vi "_CSM Scripts Colors.vi"(8 "Error In":errorcluster caption="error in (no error)", 11 "Value":string) -> (0 "error out":errorcluster, 3 "Array":T1(array[cluster]))   [LabVIEW 2017]
uses:
  _Shared/CSM Shared.lvlib
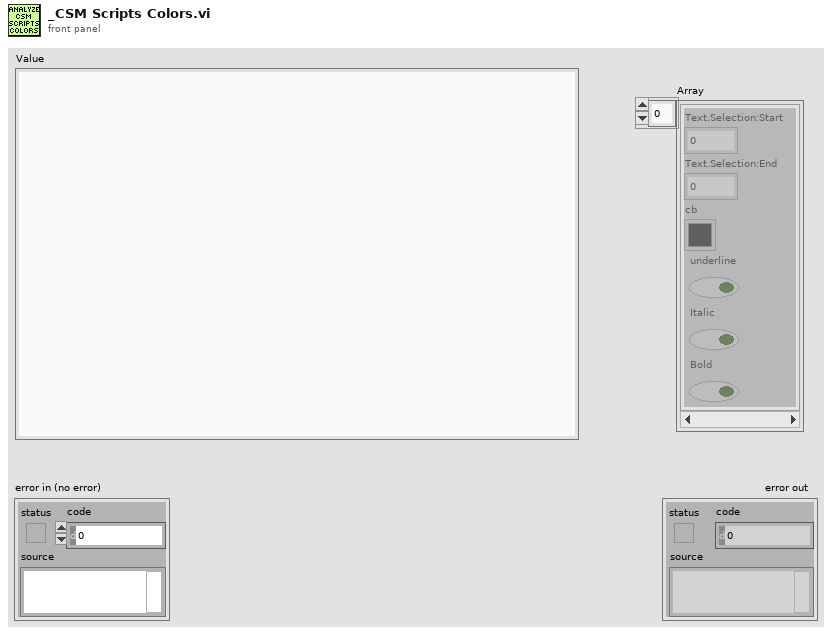
[diagram p1: front panel]
types:
  T1 = cluster{"Text.Selection:Start":u32, "Text.Selection:End":u32, "cb":u32, "underline":bool, "Italic":bool, "Bold":bool}[]
  T2 = cluster{"Text.Selection:Start":u32, u32, u32, bool, bool, bool}
  T3 = cluster{"Text.Selection:Start":u32, u32, u32, bool, bool, bool}[]
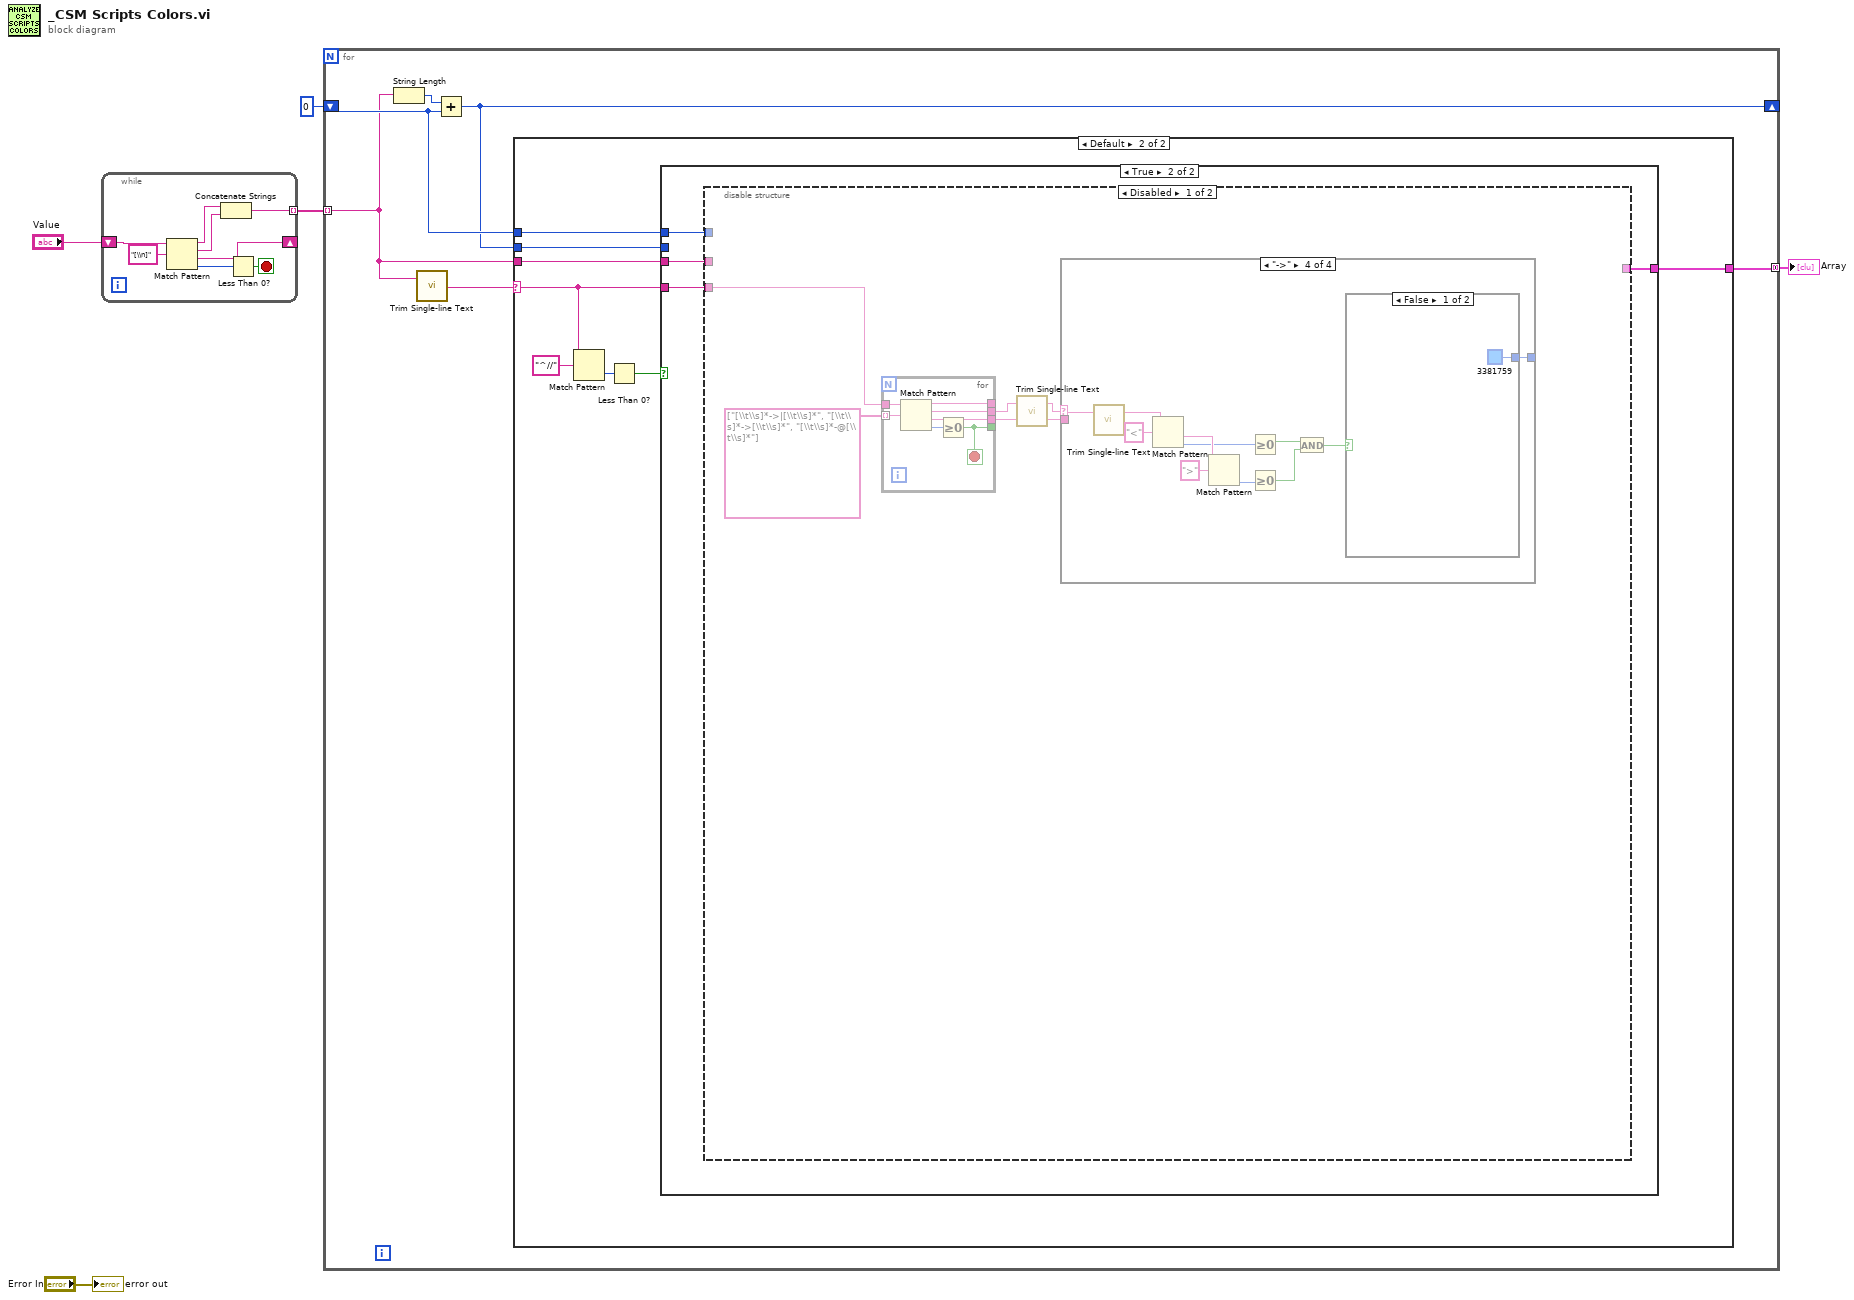
[diagram p0: block diagram]
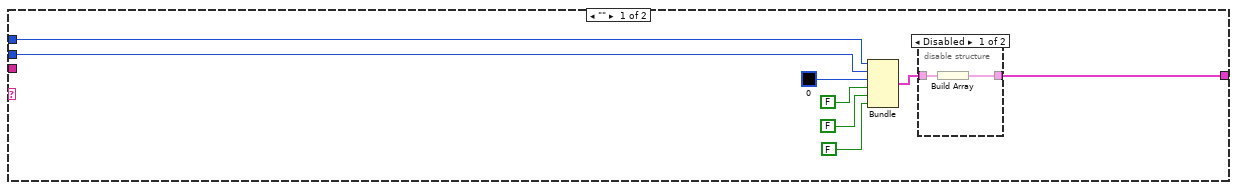
[diagram p2: hidden frame]
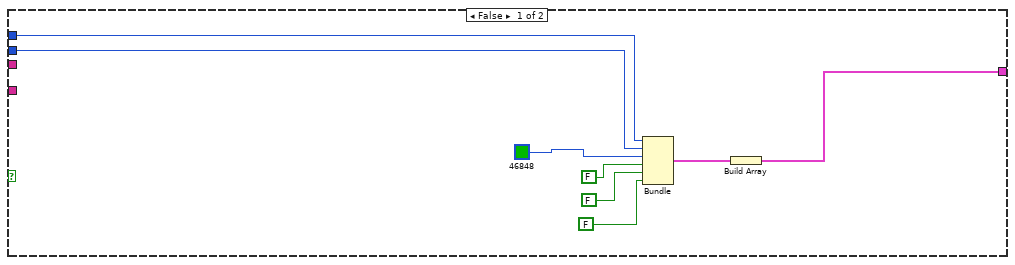
[diagram p4: hidden frame]
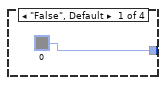
[diagram p5: hidden frame]
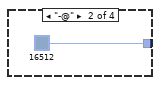
[diagram p6: hidden frame]
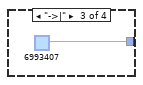
[diagram p7: hidden frame]
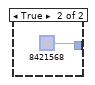
[diagram p8: hidden frame]
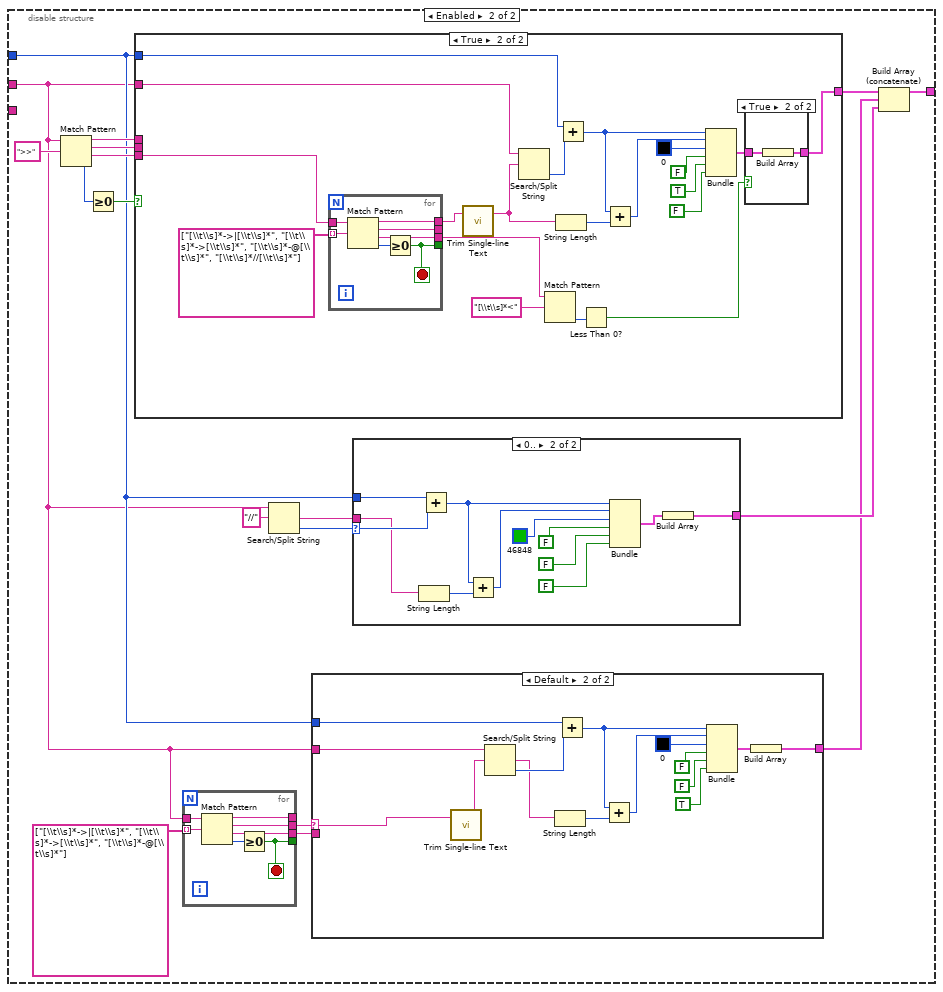
[diagram p9: hidden frame]
diagram:
  n1 = while {
    shift-right: [w12] -> _
    shift-left: "Value" -> [w13]
    tunnel: [w8] -> w5 mode=indexing
    stop <- w6 stop-if-true
    n2 = Match Pattern(string=w13, regular expression="[\\n]") -> (before substring=w10:string, match substring=w9:string, after substring=w12:string, offset past match=w7:i32)  [unwired: 1 in]
    n3 = Concatenate Strings(w10, w9) -> (w8:string)
    n4 = Less Than 0?(x=w7) -> (x < 0?=w6:bool)
  }
  n5 = for {
    tunnel: w5 -> [w14] mode=indexing
    shift-right: [w16] -> _
    shift-left: u32 0 ("Text.Selection:Start") -> [w17]
    tunnel: [w15] -> w2 mode=concatenating
    n6 = String Length(string=w14) -> (length=w18:i32)
    n7 = call "Trim Single-line Text.vi"("single-line text"=w14) -> ("trimed text"=w19:string)  [unwired: 2 in]
    n8 = Add(x=w18, y=w17) -> (x+y=w16:u32)
    n9 = case shown="Default" w19 {
      selector: w19 -> [_ w35]
      tunnel: w17 -> [w27 w32]
      tunnel: w16 -> [w26 w31]
      tunnel: [w23 w30] -> w15
      tunnel: w14 -> [_ w33]
      frame "" {
        n10 = Bundle("Text.Selection:Start"=w27, w26, u32 0, FALSE, FALSE, FALSE) -> (w24:T2)  [unwired: 1 in]
        n11 = disable-structure shown="Disabled" {
          disable-tunnel: w24 -> [w29 _]
          disable-tunnel: [w28 _] -> w23
          frame Disabled {
            n12 = Build Array(w29) -> (w28:T3)
          }
          frame Enabled {
          }
        }
      }
      frame Default {
        n13 = Match Pattern(string=w35, regular expression="^//") -> (offset past match=w37:i32)  [unwired: 1 in, 3 out]
        n14 = Less Than 0?(x=w37) -> (x < 0?=w34:bool)
        n15 = case shown="True" w34 {
          tunnel: w35 -> [_ w49]
          tunnel: w33 -> [_ w48]
          tunnel: w32 -> [w44 w47]
          tunnel: w31 -> [w43 _]
          tunnel: [w41 w46] -> w30
          frame False {
            n16 = Bundle("Text.Selection:Start"=w44, w43, u32 46848, FALSE, FALSE, FALSE) -> (w42:T2)  [unwired: 1 in]
            n17 = Build Array(w42) -> (w41:T3)
          }
          frame True {
            n18 = disable-structure shown="Disabled" {
              disable-tunnel: w49 -> [w52 _]
              disable-tunnel: w48 -> [_ w78]
              disable-tunnel: w47 -> [_ w81]
              disable-tunnel: [_ w85] -> w46
              frame Disabled {
                n19 = for {
                  tunnel: w52 -> [w77]
                  tunnel: string[] ["[\\t\\s]*->|[\\t\\s]*", "[\\t\\s]*->[\\t\\s]*", "[\\t\\s]*-@[\\t\\s]*"] -> [w76] mode=indexing
                  tunnel: [w74] -> _
                  tunnel: [w73] -> _
                  tunnel: [w72] -> w53
                  tunnel: [w71] -> w50
                  stop <- w74 stop-if-true
                  n20 = Match Pattern(string=w77, regular expression=w76) -> (before substring=w73:string, match substring=w72:string, after substring=w71:string, offset past match=w75:i32)  [unwired: 1 in]
                  n21 = Greater Or Equal To 0?(x=w75) -> (x >= 0?=w74:bool)
                }
                n22 = call "Trim Single-line Text.vi"("single-line text"=w53) -> ("trimed text"=w51:string)  [unwired: 2 in]
                n23 = case shown="\"->\"" w51 {
                  tunnel: [u32 0 u32 16512 u32 6993407 w68] -> _
                  tunnel: w50 -> [_ _ _ w67]
                  frame "False", Default {
                  }
                  frame "-@" {
                  }
                  frame "->|" {
                  }
                  frame "->" {
                    n24 = call "Trim Single-line Text.vi"("single-line text"=w67) -> ("trimed text"=w66:string)  [unwired: 2 in]
                    n25 = Match Pattern(string=w66, regular expression="<") -> (after substring=w63:string, offset past match=w61:i32)  [unwired: 1 in, 2 out]
                    n26 = Match Pattern(string=w63, regular expression=">") -> (offset past match=w62:i32)  [unwired: 1 in, 3 out]
                    n27 = Greater Or Equal To 0?(x=w61) -> (x >= 0?=w60:bool)
                    n28 = Greater Or Equal To 0?(x=w62) -> (x >= 0?=w59:bool)
                    n29 = And(x=w60, y=w59) -> (x .and. y?=w58:bool)
                    n30 = case shown="False" w58 {
                      tunnel: [u32 3381759 u32 8421568] -> w68
                      frame False {
                      }
                      frame True {
                      }
                    }
                  }
                }
              }
              frame Enabled {
                n31 = Match Pattern(string=w78, regular expression=">>") -> (before substring=w94:string, match substring=w95:string, after substring=w91:string, offset past match=w92:i32)  [unwired: 1 in]
                n32 = Greater Or Equal To 0?(x=w92) -> (x >= 0?=w93:bool)
                n33 = case shown="True" w93 {
                  tunnel: w91 -> [_ w149]
                  tunnel: w94 -> [_ _]
                  tunnel: w95 -> [_ _]
                  tunnel: w78 -> [_ w147]
                  tunnel: w81 -> [_ w145]
                  tunnel: [_ w137] -> w89
                  frame False {
                  }
                  frame True {
                    n34 = for {
                      tunnel: w149 -> [w158]
                      tunnel: string[] ["[\\t\\s]*->|[\\t\\s]*", "[\\t\\s]*->[\\t\\s]*", "[\\t\\s]*-@[\\t\\s]*", "[\\t\\s]*//[\\t\\s]*"] -> [w157] mode=indexing
                      tunnel: [w155] -> _
                      tunnel: [w154] -> w142
                      tunnel: [w153] -> _
                      tunnel: [w152] -> w134
                      stop <- w155 stop-if-true
                      n35 = Match Pattern(string=w158, regular expression=w157) -> (before substring=w154:string, match substring=w153:string, after substring=w152:string, offset past match=w156:i32)  [unwired: 1 in]
                      n36 = Greater Or Equal To 0?(x=w156) -> (x >= 0?=w155:bool)
                    }
                    n37 = call "Trim Single-line Text.vi"("single-line text"=w142) -> ("trimed text"=w130:string)  [unwired: 2 in]
                    n38 = Search/Split String(string=w147, search string/char (-)=w130) -> (offset of match=w146:i32)  [unwired: 1 in, 2 out]
                    n39 = Match Pattern(string=w134, regular expression="[\\t\\s]*<") -> (offset past match=w132:i32)  [unwired: 1 in, 3 out]
                    n40 = String Length(string=w130) -> (length=w141:i32)
                    n41 = Add(x=w145, y=w146) -> (x+y=w140:u32)
                    n42 = Less Than 0?(x=w132) -> (x < 0?=w131:bool)
                    n43 = Add(x=w140, y=w141) -> (x+y=w139:u32)
                    n44 = Bundle(w140, w139, u32 0, FALSE, TRUE, FALSE) -> (w138:cluster{u32, u32, u32, bool, bool, bool})  [unwired: 1 in]
                    n45 = case shown="True" w131 {
                      tunnel: w138 -> [_ w151]
                      tunnel: [_ w150] -> w137
                      frame False {
                      }
                      frame True {
                        n46 = Build Array(w151) -> (w150:cluster{u32, u32, u32, bool, bool, bool}[])
                      }
                    }
                  }
                }
                n47 = for {
                  tunnel: w78 -> [w117]
                  tunnel: string[] ["[\\t\\s]*->|[\\t\\s]*", "[\\t\\s]*->[\\t\\s]*", "[\\t\\s]*-@[\\t\\s]*"] -> [w116] mode=indexing
                  tunnel: [w114] -> _
                  tunnel: [w113] -> _
                  tunnel: [w112] -> w82
                  tunnel: [w111] -> w79
                  stop <- w114 stop-if-true
                  n48 = Match Pattern(string=w117, regular expression=w116) -> (before substring=w113:string, match substring=w112:string, after substring=w111:string, offset past match=w115:i32)  [unwired: 1 in]
                  n49 = Greater Or Equal To 0?(x=w115) -> (x >= 0?=w114:bool)
                }
                n50 = Search/Split String(string=w78, search string/char (-)="//" ("regular expression")) -> (match + rest of string=w86:string, offset of match=w87:i32)  [unwired: 1 in, 1 out]
                n51 = case shown="Default" w82 {
                  selector: w82 -> [_ w100]
                  tunnel: w78 -> [_ w101]
                  tunnel: w81 -> [_ w97]
                  tunnel: [_ w96] -> w80
                  tunnel: w79 -> [_ _]
                  frame "" {
                  }
                  frame Default {
                    n52 = call "Trim Single-line Text.vi"("single-line text"=w100) -> ("trimed text"=w99:string)  [unwired: 2 in]
                    n53 = Search/Split String(string=w101, search string/char (-)=w99) -> (match + rest of string=w98:string, offset of match=w110:i32)  [unwired: 1 in, 1 out]
                    n54 = String Length(string=w98) -> (length=w107:i32)
                    n55 = Add(x=w97, y=w110) -> (x+y=w106:u32)
                    n56 = Add(x=w106, y=w107) -> (x+y=w105:u32)
                    n57 = Bundle(w106, w105, u32 0, FALSE, FALSE, TRUE) -> (w104:cluster{u32, u32, u32, bool, bool, bool})  [unwired: 1 in]
                    n58 = Build Array(w104) -> (w96:cluster{u32, u32, u32, bool, bool, bool}[])
                  }
                }
                n59 = case shown="0.." w87 {
                  selector: w87 -> [_ w124]
                  tunnel: w86 -> [_ w123]
                  tunnel: w81 -> [_ w122]
                  tunnel: [_ w121] -> w84
                  frame Default {
                  }
                  frame 0.. {
                    n60 = String Length(string=w123) -> (length=w126:i32)
                    n61 = Add(x=w122, y=w124) -> (x+y=w127:u32)
                    n62 = Add(x=w127, y=w126) -> (x+y=w128:u32)
                    n63 = Bundle(w127, w128, u32 46848, FALSE, FALSE, FALSE) -> (w129:cluster{u32, u32, u32, bool, bool, bool})  [unwired: 1 in]
                    n64 = Build Array(w129) -> (w121:cluster{u32, u32, u32, bool, bool, bool}[])
                  }
                }
                n65 = Build Array (concatenate)(w89, w80, w84) -> (w85:cluster{u32, u32, u32, bool, bool, bool}[])
              }
            }
          }
        }
      }
    }
  }
  "Array" <- w2
  "error out" <- "Error In"
